vi "ALTS-2015 Read a Section Values from INI File (String).vi"(6 "Data Type":string, 7 "Section":string="Power Supply Tap Setting", 8 "error in (no error)":errorcluster, 11 "INI File Path":path) -> (0 "error out":errorcluster, 2 "Key Values":string[](array[string]), 3 "Key Names":string[](array[string]))   [LabVIEW 2013]
doc: "Reads all the values of the specified section and gives out along with the key names. If there is any empty line in the section, it is ignored.\n\n- Senthil."
uses:
  <vilib>/Utility/config.llb/Read Key (String).vi
  <vilib>/Utility/config.llb/NI_LVConfig.lvlib
panel:
  # "Inputs"
  # "Outputs"
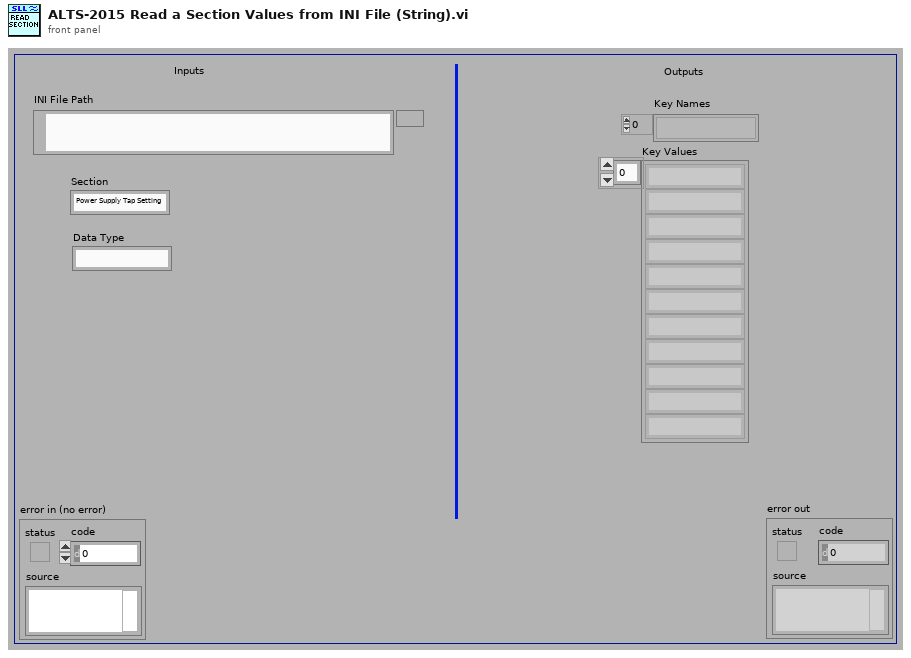
[diagram p1: front panel]
types:
  T1 = typedef "NI_LVConfig.lvlib/Config Data RefNum.ctl" = refnum<k1>
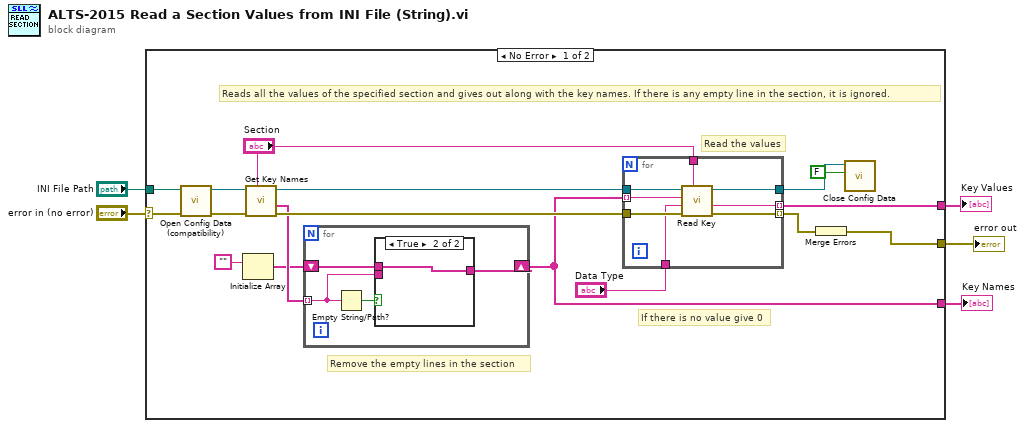
[diagram p0: block diagram]
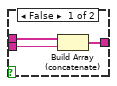
[diagram p2: hidden frame]
diagram:
  n1 = case shown="No Error" "error in (no error)" {
    selector: "error in (no error)" -> [w21 w39]
    tunnel: [w8 w39] -> w4
    tunnel: "INI File Path" -> [w22 _]
    tunnel: [w15 _] -> w2
    tunnel: [w10 _] -> w1
    frame No Error {
      # "If there is no value give 0"
      # "Read the values"
      # "Remove the empty lines in the section"
      # "Reads all the values of the specified section and gives out along with the key names. If there is any empty line in the section, it is ignored."
      n2 = call <vilib>:"Open Config Data (compatibility).vi"("error in (no error)"=w21, "configuration file path"=w22) -> ("error out"=w20:errorcluster, "refnum"=w19:T1)  [unwired: 7 in, 1 out]
      n3 = Initialize Array("") -> (w11:string[])  [unwired: 1 in]
      n4 = call <vilib>:"Get Key Names.vi"("section"="Section", "error in (no error)"=w20, "refnum"=w19) -> ("error out"=w17:errorcluster, "key names"=w13:string[], "refnum out"=w16:T1)  [unwired: 5 in, 1 out]
      n5 = for {
        shift-right: [w23] -> w10
        shift-left: w11 -> [w25]
        tunnel: w13 -> [w24] mode=indexing
        n6 = Empty String/Path?(string/path=w24) -> (empty?=w26:bool)
        n7 = case shown="True" w26 {
          tunnel: w25 -> [w29 w30]
          tunnel: w24 -> [w28 _]
          tunnel: [w27 w30] -> w23
          frame False {
            n8 = Build Array (concatenate)(w29, w28) -> (w27:string[])
          }
          frame True {
          }
        }
      }
      n9 = for {
        tunnel: w17 -> [w38]
        tunnel: w16 -> [w37]
        tunnel: w10 -> [w36] mode=indexing
        tunnel: "Section" -> [w35]
        tunnel: "Data Type" -> [w34]
        tunnel: [w33] -> w15 mode=indexing
        tunnel: [w32] -> w9 mode=indexing
        tunnel: [w31] -> w14
        n10 = call-poly <vilib>:"Read Key.vi"("section"=w35, "error in (no error)"=w38, "default value"=w34, "key"=w36, "refnum"=w37) -> ("error out"=w32:errorcluster, "value"=w33:string, "refnum out"=w31:T1)  [unwired: 3 in, 1 out]
      }
      n11 = Merge Errors(w9) -> (w8:errorcluster)
      n12 = call <vilib>:"Close Config Data.vi"("write file if changed (T)"=FALSE ("write configuration file? (T)"), "refnum"=w14) -> ()  [unwired: 8 in, 2 out]
    }
    frame Error {
    }
  }
  "error out" <- w4
  "Key Values" <- w2
  "Key Names" <- w1
